vi "Main_Set_Field_v1.vi"(6 "stop":bool, 8 "error in (no error)":errorcluster, 9 "Field in Gauss":i32, 10 "Limit":bool, 11 "VISA session":refnum<visa-resource-name>="GPIB0::1::INSTR") -> (0 "error out":errorcluster)   [LabVIEW 2010]
panel:
  out "field out":dbl format="%#_4g"
  out "response out":string
  out "field (kGauss)":dbl=-1.0 format="%.4f"
  out "Action":string
  # "Created by Nusran. Dec 2018"
  # "Upper"
  # "Lower"
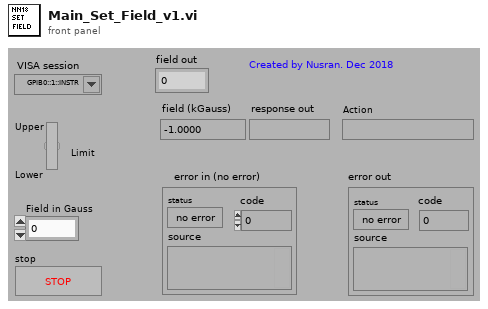
[diagram p1: front panel]
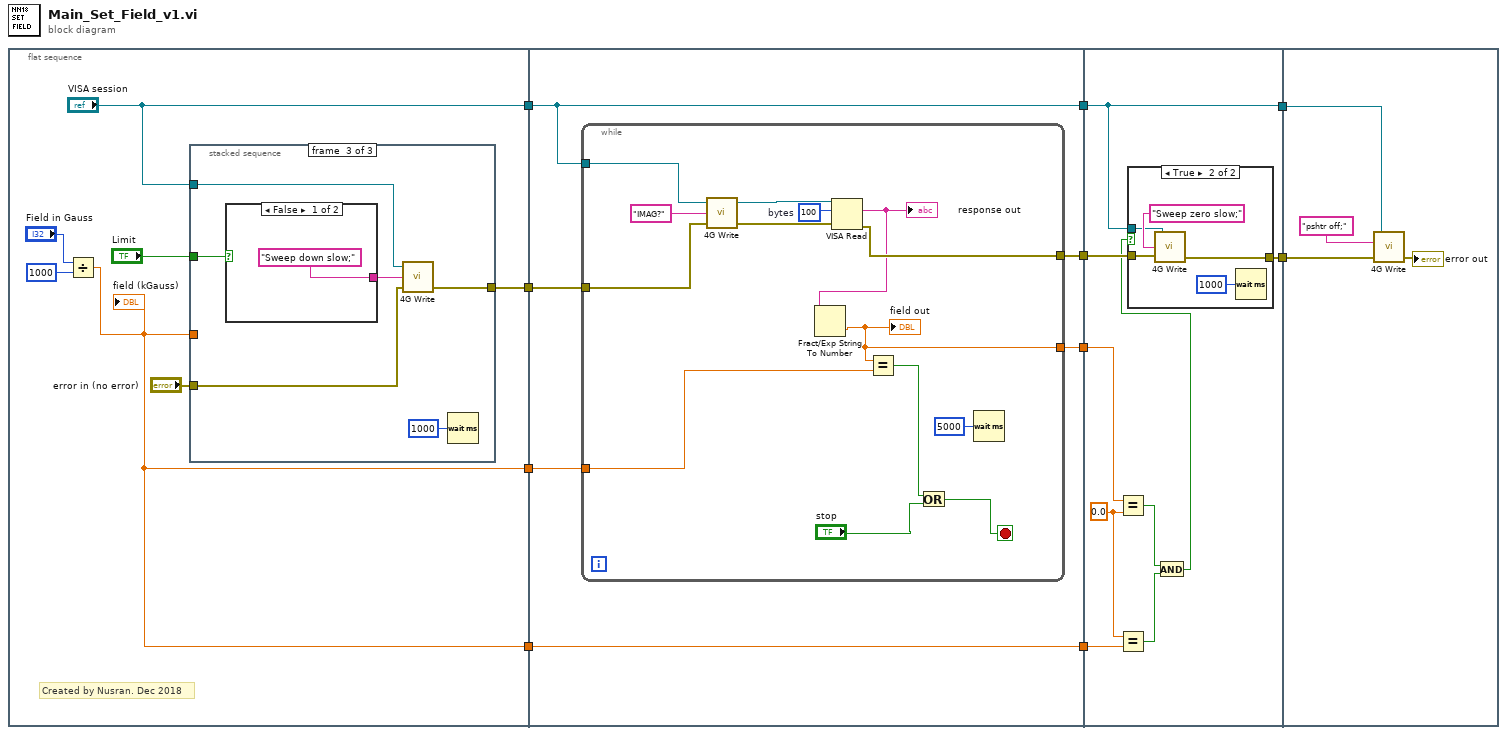
[diagram p0: block diagram]
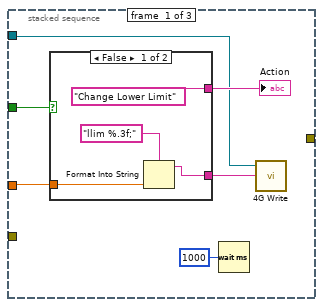
[diagram p2: hidden frame]
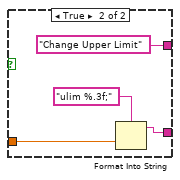
[diagram p3: hidden frame]
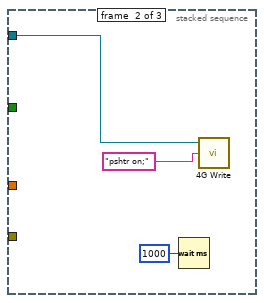
[diagram p4: hidden frame]
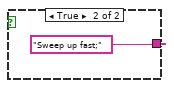
[diagram p5: hidden frame]
diagram:
  n1 = flat-sequence {
    tunnel: [w15] -> w10
    tunnel: ["VISA session"] -> w9
    tunnel: [w11] -> w6
    tunnel: [w11] -> w1
    tunnel: w10 -> [w48]
    tunnel: w9 -> [w46]
    tunnel: [w47] -> w8
    tunnel: [w46] -> w7
    tunnel: w6 -> [w45]
    tunnel: [w44] -> w3
    tunnel: [w43] -> w2
    tunnel: w1 -> [w43]
    tunnel: w8 -> [w71]
    tunnel: w7 -> [w69]
    tunnel: [w69] -> w5
    tunnel: [w70] -> w4
    tunnel: w3 -> [w68]
    tunnel: w2 -> [w67]
    tunnel: w5 -> [w79]
    tunnel: w4 -> [w78]
    frame #0 {
      # "Created by Nusran. Dec 2018"
      n2 = Divide(x="Field in Gauss", y=1000) -> (x/y=w11:dbl)
      "field (kGauss)" <- w11
      n3 = stacked-sequence {
        tunnel: w11 -> [w21 _ _]
        tunnel: "Limit" -> [w20 _ w40]
        tunnel: "VISA session" -> [w18 w33 w38]
        tunnel: "error in (no error)" -> [_ _ w36]
        tunnel: [_ _ w35] -> w15
        frame #0 {
          n4 = case shown="False" w20 {
            tunnel: ["Change Lower Limit" "Change Upper Limit"] -> w23
            tunnel: w21 -> [w25 w29]
            tunnel: [w24 w28] -> w22
            frame False {
              n5 = Format Into String(format string="llim %.3f;", w25) -> (resulting string=w24:string)  [unwired: 2 in, 1 out]
            }
            frame True {
              n6 = Format Into String(format string="ulim %.3f;", w29) -> (resulting string=w28:string)  [unwired: 2 in, 1 out]
            }
          }
          "Action" <- w23
          n7 = Wait (ms)(milliseconds to wait=u32 1000) -> ()  [unwired: 1 out]
          n8 = call "4G Write.vi"("write buffer (\"\")"=w22, "VISA session"=w18) -> ()  [unwired: 1 in, 3 out]
        }
        frame #1 {
          n9 = Wait (ms)(milliseconds to wait=u32 1000) -> ()  [unwired: 1 out]
          n10 = call "4G Write.vi"("write buffer (\"\")"="pshtr on;", "VISA session"=w33) -> ()  [unwired: 1 in, 3 out]
        }
        frame #2 {
          n11 = case shown="False" w40 {
            tunnel: ["Sweep down slow;" "Sweep up fast;"] -> w39
            frame False {
            }
            frame True {
            }
          }
          n12 = call "4G Write.vi"("error in (no error)"=w36, "write buffer (\"\")"=w39, "VISA session"=w38) -> ("error out"=w35:errorcluster)  [unwired: 2 out]
          n13 = Wait (ms)(milliseconds to wait=u32 1000) -> ()  [unwired: 1 out]
        }
      }
    }
    frame #1 {
      n14 = while {
        tunnel: w48 -> [w57]
        tunnel: w46 -> [w56]
        tunnel: [w55] -> w47
        tunnel: w45 -> [w53]
        tunnel: [w49] -> w44
        stop <- w50 stop-if-true
        w59 = u32 100  # bytes
        n15 = call "4G Write.vi"("error in (no error)"=w57, "write buffer (\"\")"="IMAG?", "VISA session"=w56) -> ("error out"=w60:errorcluster, "dup VISA session"=w61:refnum<visa-resource-name>)  [unwired: 1 out]
        n16 = VISA Read(VISA resource name=w61, byte count=w59, error in (no error)=w60) -> (read buffer=w54:string, error out=w55:errorcluster)  [unwired: 2 out]
        "response out" <- w54
        n17 = Fract/Exp String To Number(string=w54) -> (number=w49:dbl)  [unwired: 3 in, 1 out]
        "field out" <- w49
        n18 = Equal?(x=w49, y=w53) -> (x = y?=w52:bool)
        n19 = Or(x=w52, y="stop") -> (x .or. y?=w50:bool)
        n20 = Wait (ms)(milliseconds to wait=u32 5000) -> ()  [unwired: 1 out]
      }
    }
    frame #2 {
      w66 = 0.0 ("y")
      n21 = Equal?(x=w68, y=w66) -> (x = y?=w65:bool)
      n22 = Equal?(x=w66, y=w67) -> (x = y?=w64:bool)
      n23 = And(x=w65, y=w64) -> (x .and. y?=w63:bool)
      n24 = case shown="True" w63 {
        tunnel: w71 -> [w72 w76]
        tunnel: [w72 w75] -> w70
        tunnel: w69 -> [_ w74]
        frame False {
        }
        frame True {
          n25 = call "4G Write.vi"("error in (no error)"=w76, "write buffer (\"\")"="Sweep zero slow;", "VISA session"=w74) -> ("error out"=w75:errorcluster)  [unwired: 2 out]
          n26 = Wait (ms)(milliseconds to wait=u32 1000) -> ()  [unwired: 1 out]
        }
      }
    }
    frame #3 {
      n27 = call "4G Write.vi"("error in (no error)"=w78, "write buffer (\"\")"="pshtr off;", "VISA session"=w79) -> ("error out"=→"error out":errorcluster)  [unwired: 2 out]
    }
  }
